vi "proc_DLL_path.vi"(8 "error in":errorcluster, 11 "path in":path) -> (0 "error out":errorcluster, 3 "path out":path)   [LabVIEW 2011]
doc: "Sets and returns lv_process DLL path. If not initialized lv_process VI's expects DLL in appliaction folder."
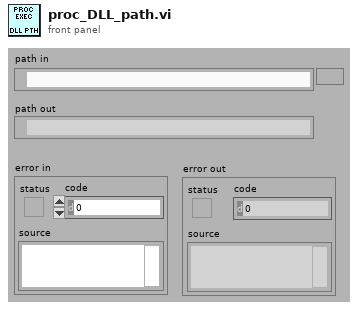
[diagram p1: front panel]
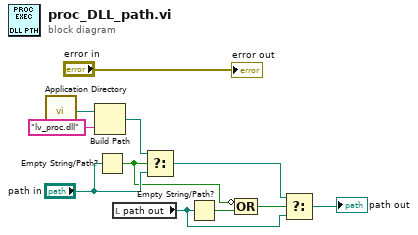
[diagram p0: block diagram]
diagram:
  n1 = call <vilib>:"Application Directory.vi"() -> ("Application Directory"=w9:path)
  n2 = Build Path(base path=w9, name or relative path="lv_proc.dll") -> (appended path=w10:path)
  n3 = Empty String/Path?(string/path="path in") -> (empty?=w6:bool)
  n4 = local read "path out"() -> (w2:path)
  n5 = Select(t=w10, s=w6, f="path in") -> (s? t:f=w3:path)
  n6 = Empty String/Path?(string/path=w2) -> (empty?=w7:bool)
  n7 = Compound Arithmetic op=OR(invert w6, w7) -> (w5:bool)
  n8 = Select(t=w3, s=w5, f=w2) -> (s? t:f=→"path out":path)
  "error out" <- "error in"
